vi "topvi_puzzle.vi"() -> ()   [LabVIEW 2014]
panel:
  in  "stop":bool
  out "Used Time(s)":dbl caption="Elapsed Time (s)"
  out "Game Array":picture[][](array[picture])
  in  "marvel":T1
  in  "Difficulty":i32(slide) scale=1.0..3.0
  # "step1.選擇難易度(2*2、3*3、4*4)"
  # "step2.選擇類型"
  # "step3.執行"
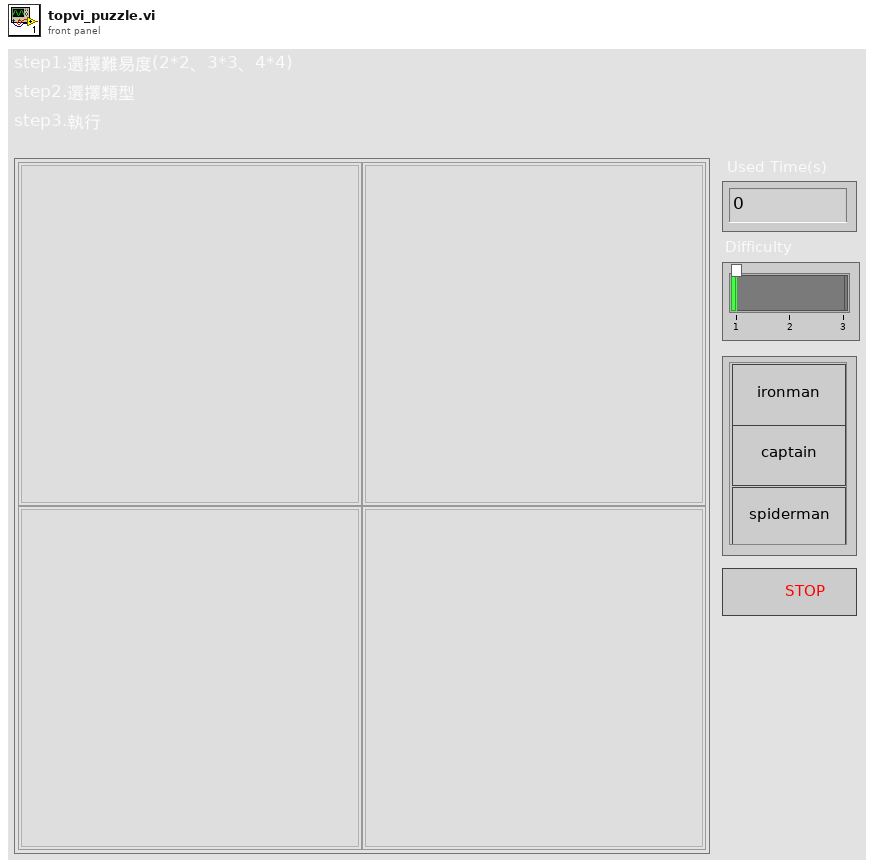
[diagram p1: front panel]
types:
  T1 = cluster{"Blank Button 2":bool, "Blank Button 3":bool, "Blank Button":bool}
  T2 = typedef "imagedata.ctl" = cluster{"image type":i32, "image depth":i32, "image":u8[], "mask":u8[], "colors":u32[], "Rectangle":cluster{"left":i16, "top":i16, "right":i16, "bottom":i16}}
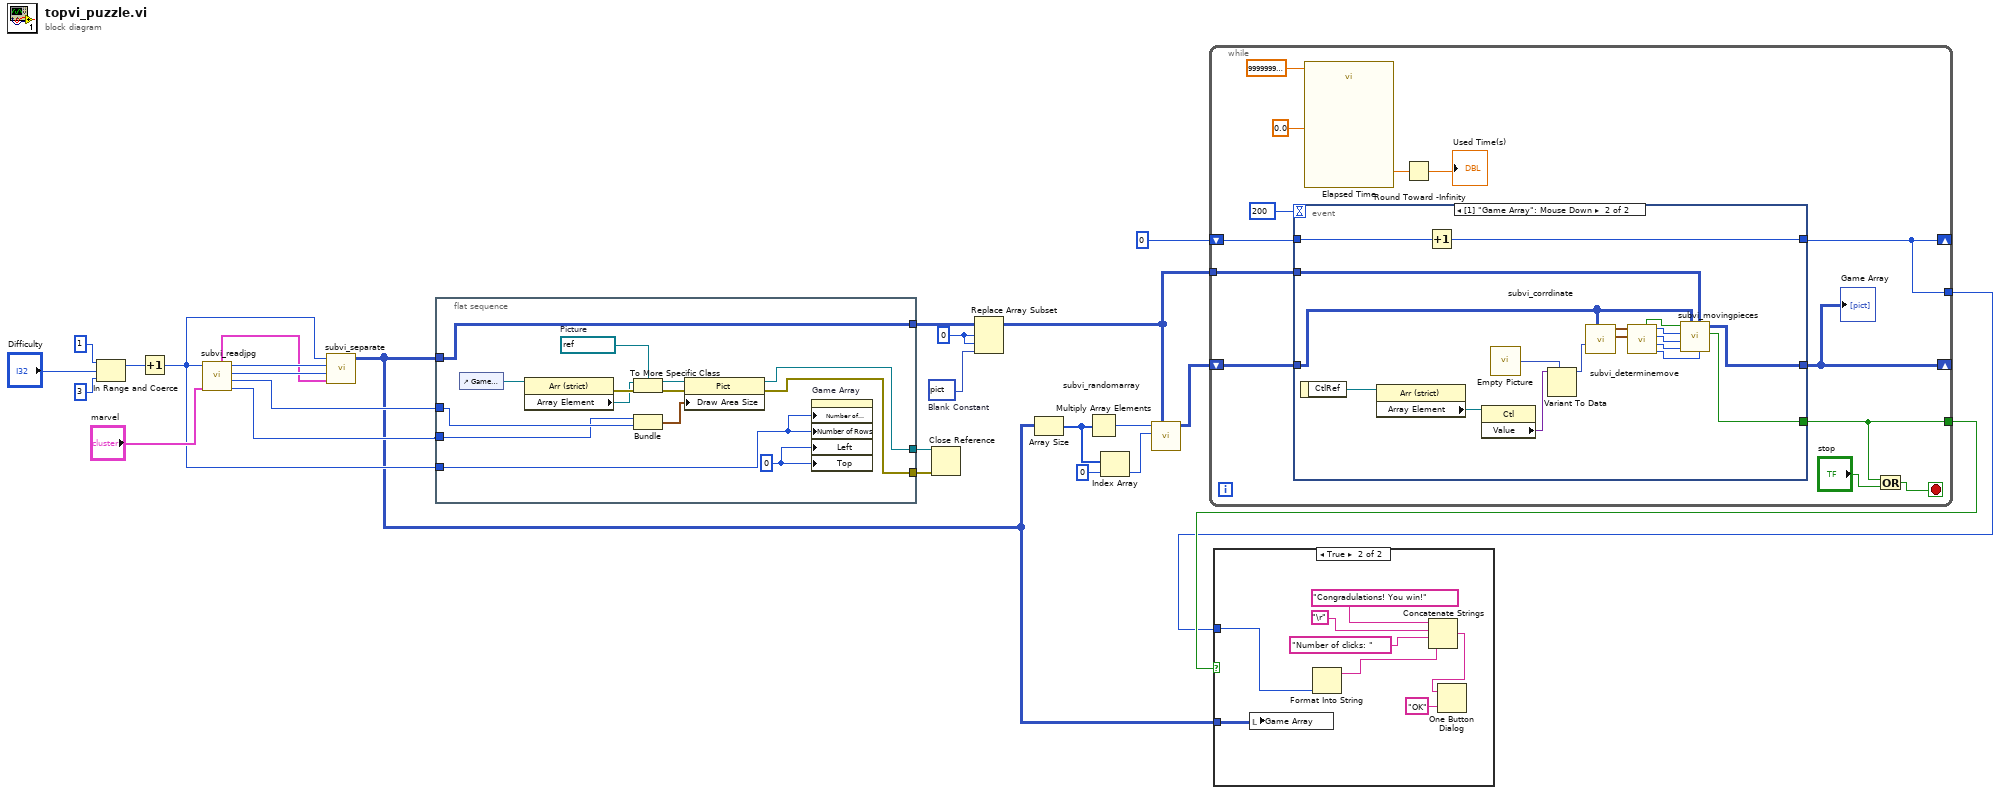
[diagram p0: block diagram]
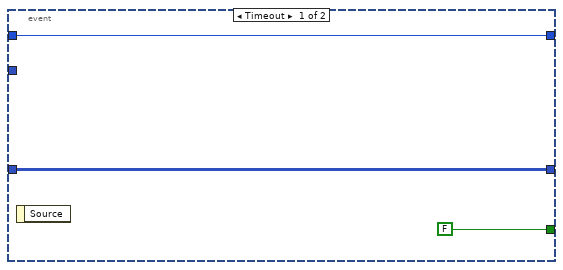
[diagram p3: hidden frame]
diagram:
  w12 = 0 ("index (row)")
  w5 = picture data[5B]  # Blank Constant
  n1 = In Range and Coerce(upper limit=1, x="Difficulty", lower limit=3) -> (coerced(x)=w6:i32)  [unwired: 1 out]
  n2 = Increment(x=w6) -> (x+1=w19:i32)
  n3 = call "subvi_readjpg.vi"("Cluster"="marvel", "length"=w19) -> ("image size y"=w17:i32, "image size x"=w18:i32, "image subset y"=w21:i32, "image subset x"=w22:i32, "image data"=w20:T2)  [unwired: 5 in]
  n4 = call "subvi_separate.vi"("image data"=w20, "subset y"=w21, "subset x"=w22, "length"=w19) -> ("separated image array"=w10:picture[][])  [unwired: 7 in]
  n5 = flat-sequence {
    tunnel: [w27] -> w23
    tunnel: [w28] -> w24
    tunnel: w19 -> [w33]
    tunnel: w18 -> [w32]
    tunnel: w17 -> [w31]
    tunnel: w10 -> [w29]
    tunnel: [w29] -> w11
    frame #0 {
      w35 = refnum<vi> refnum  # Picture
      w40 = 0
      n6 = control-ref of="Game Array"() -> (w39:refnum<vi>)
      n7 = property on="Property Node" class="Arr (strict)"(reference=w39) -> (error out=w38:errorcluster, "Array Element"=w36:refnum<vi>)  [unwired: 1 in, 1 out]
      n8 = To More Specific Class(target class=w35, reference=w36, error in=w38) -> (specific class reference=w34:refnum<vi>, error out=w37:errorcluster)
      n9 = Bundle("image size y"=w31, "image size x"=w32) -> (w30:cluster{"image size y":i32, "image size x":i32})  [unwired: 1 in]
      n10 = property class="Pict"(reference=w34, error in=w37, "Draw Area Size"=w30) -> (reference out=w28:refnum<vi>, error out=w27:errorcluster)
      n11 = property on="Game Array" class="Arr (strict)"("Number of Columns"=w33, "Number of Rows"=w33, "Left"=w40, "Top"=w40) -> ()  [unwired: 2 in, 2 out]
    }
  }
  n12 = Close Reference(reference=w24, error in (no error)=w23) -> ()  [unwired: 1 out]
  n13 = Replace Array Subset(array=w11, new element=w5, index (row)=w12, index (col)=w12) -> (w2:picture[][])
  n14 = Array Size(array=w10) -> (size(s)=w16:i32[])
  n15 = Multiply Array Elements(1:w16) -> (0:w4:i32)
  n16 = Index Array(array=w16, index=0) -> (element=w3:i32)
  n17 = call "subvi_randomarray.vi"("original image"=w2, "Width/Height"=w3, "Element number"=w4) -> ("random array"=w1:picture[][])  [unwired: 8 in]
  n18 = while {
    shift-right: [w47] -> _
    shift-left: 0 ("index (row)") -> [w52]
    shift-right: [w42] -> _
    shift-left: w1 -> [w50]
    tunnel: w2 -> [w51]
    tunnel: [w41] -> w14
    tunnel: [w47] -> w13
    stop <- w49 stop-if-true
    n19 = event shown="[1] \"Game Array\": Mouse Down" {
      selector: _ -> [_ _]
      dyn-events: _ -> [_ _]
      timeout: 200 -> [_ _]
      tunnel: w52 -> [w56 w63]
      tunnel: w51 -> [_ w60]
      tunnel: w50 -> [w55 w61]
      tunnel: [w56 w62] -> w47
      tunnel: [w55 w59] -> w42
      tunnel: [FALSE w58] -> w41
      event Timeout {
        n20 = event-data() -> ()  [unwired: 1 in, 1 out]
      }
      event "Game Array": Mouse Down {
        n21 = event-data() -> ("CtlRef"=w57:refnum<vi>)  [unwired: 1 in]
        n22 = property class="Arr (strict)"(reference=w57) -> ("Array Element"=w74:refnum<vi>)  [unwired: 1 in, 2 out]
        n23 = Increment(x=w63) -> (x+1=w62:i32)
        n24 = property class="Ctl"(reference=w74) -> ("Value"=w73:variant)  [unwired: 1 in, 2 out]
        n25 = call "Empty Picture"() -> ("empty picture"=w72:picture)
        n26 = Variant To Data(type=w72, Variant=w73) -> (data=w71:picture)  [unwired: 1 in, 1 out]
        n27 = call "subvi_corrdinate.vi"("current puzzle"=w61, "2D Picture"=w71) -> ("white location"=w69:cluster{i32, i32}, "piece location"=w70:cluster{i32, i32})  [unwired: 8 in]
        n28 = call "subvi_determinemove.vi"("white lacation"=w69, "puzzle lacation"=w70) -> ("Upper White Row Position"=w64:i32, "Current Peice Column"=w65:i32, "Current Peice Row"=w66:i32, "Lower White Column Position"=w67:i32, "Allow Peice Movement"=w68:bool)  [unwired: 5 in]
        n29 = call "subvi_movingpieces.vi"("Upper White Row"=w64, "solved puzzle"=w60, "current puzzle state"=w61, "Current Selected Peice Column"=w65, "Current Selected Peice Row"=w66, "Lower White  Column"=w67, "Allow Peice Movement"=w68) -> ("Puzzle Finished"=w58:bool, "updated image array"=w59:picture[][])  [unwired: 3 in]
      }
    }
    "Game Array" <- w42
    n30 = call "Elapsed Time"("Time Target (s)"=99999999999999.0, "Set Start Time (s)"=0.0) -> ("Elapsed Time (s)"=w45:dbl)  [unwired: 10 in, 7 out]
    n31 = Round Toward -Infinity(1:w45) -> (0:→"Used Time(s)":dbl)
    n32 = Or(x=w41, y="stop") -> (x .or. y?=w49:bool)
  }
  n33 = case shown="True" w14 {
    tunnel: w10 -> [_ w76]
    tunnel: w13 -> [_ w75]
    frame False {
    }
    frame True {
      n34 = local write "Game Array"(w76) -> ()
      n35 = Format Into String(w75) -> (resulting string=w82:string)  [unwired: 3 in, 1 out]
      n36 = Concatenate Strings("Congradulations! You win!", "\r", "Number of clicks: ", w82) -> (w78:string)
      n37 = One Button Dialog(message=w78, button name ("OK")="OK") -> ()  [unwired: 1 out]
    }
  }
